vi "CANOpen_Check_Node_State.vi"(6 "Start NMT":bool, 8 "error in":errorcluster, 10 "Nodes":T2[](array[typedef]) {"NMT"."Node init static SDO state" items=["start remote node"=1, "enter pre-operational"=128]; "NMT"."Node run state" items=["start remote node"=1, "stop remote node"=2, "enter pre-operational"=128, "reset node"=129, "reset communication"=130]; "Dynamic SDOs"."Sub-Index (0)" format="%.0x"; "Dynamic SDOs"."Object Index" format="%.0x"; "Dynamic SDOs"."Block Data" format="%.0x"; "RPDOs"."PDO Channel" items=["PDO 1", "PDO 2", "PDO 3", "PDO 4"]; "RPDOs"."Parameters"."Bit Offset" max=8 step=1; "RPDOs"."Parameters"."Byte Offset" max=8 step=1; "TPDOs"."PDO Channel" items=["PDO 1", "PDO 2", "PDO 3", "PDO 4"]; "TPDOs"."Parameters"."Bit Offset" max=8 step=1; "TPDOs"."Parameters"."Byte Offset" max=8 step=1; "SDOs"."Sub-Index (0)" format="%.0x"; "SDOs"."Object Index" format="%.0x"; "SDOs"."Block Data" format="%.0x"}, 11 "interface object":refnum<k20>) -> (0 "error out":errorcluster, 2 "States":u16[](array[ring]) items=["unknown"=1, "bootup"=0, "stopped"=4, "operational"=5, "pre-operational"=127, "connection lost"=128], 3 "interface object out":refnum<k20>, 5 "Security Ref":T1)   [LabVIEW 2021, in "CANOpen Addon Engine.lvlib"]
uses:
  CANOpen Addon Engine.lvlib
  SubVIS/CANOpen_Node Message Settings.ctl
  Shared/CANOpen_PDO Settings.ctl
  Shared/CANOpen_PDO Parameter Settings.ctl
  Shared/CANOpen_PDO Data Type.ctl
  Shared/CANopen Byte Order.ctl
  Shared/CANOpen_SDO Settings.ctl
  SubVIS/CANOpen_NMT Settings.ctl
  Shared/CanOpen_NMT_Config.ctl
  Shared/CanOpen_NMT_Static detect.ctl
  CANOpen_HB_NG_EM Refs.ctl
  <vilib>/CANopenLib/CANOPEN.llb/CANopen Emergency Create.vi
  <vilib>/CANopenLib/CANOPEN.llb/CANopen SDO Create.vi
  <vilib>/CANopenLib/CANOPEN.llb/CANopen SDO Write [U16].vi
  <vilib>/CANopenLib/CANOPEN.llb/CANopen SDO Write [U8].vi
  <vilib>/CANopenLib/CANOPEN.llb/CANopen SDO Close.vi
  <vilib>/CANopenLib/CANOPEN.llb/CANopen Node Guarding Create.vi
  <vilib>/CANopenLib/CANOPEN.llb/CANopen Node Guarding State Read.vi
  <vilib>/CANopenLib/CANOPEN.llb/CANopen Heartbeat Create.vi
  <vilib>/CANopenLib/CANOPEN.llb/CANopen Heartbeat State Read.vi
  <resource>/objmgr/CANopenNodeGuard.rc
  <resource>/objmgr/CANopenHeartbeat.rc
  <resource>/objmgr/CANopenEmergency.rc
  Shared/CANOpen Addon Shared.lvlib
panel:
  out "Timestamp":timestamp
  # "LSB"
  # "MSB"
  # "LSB"
  # "MSB"
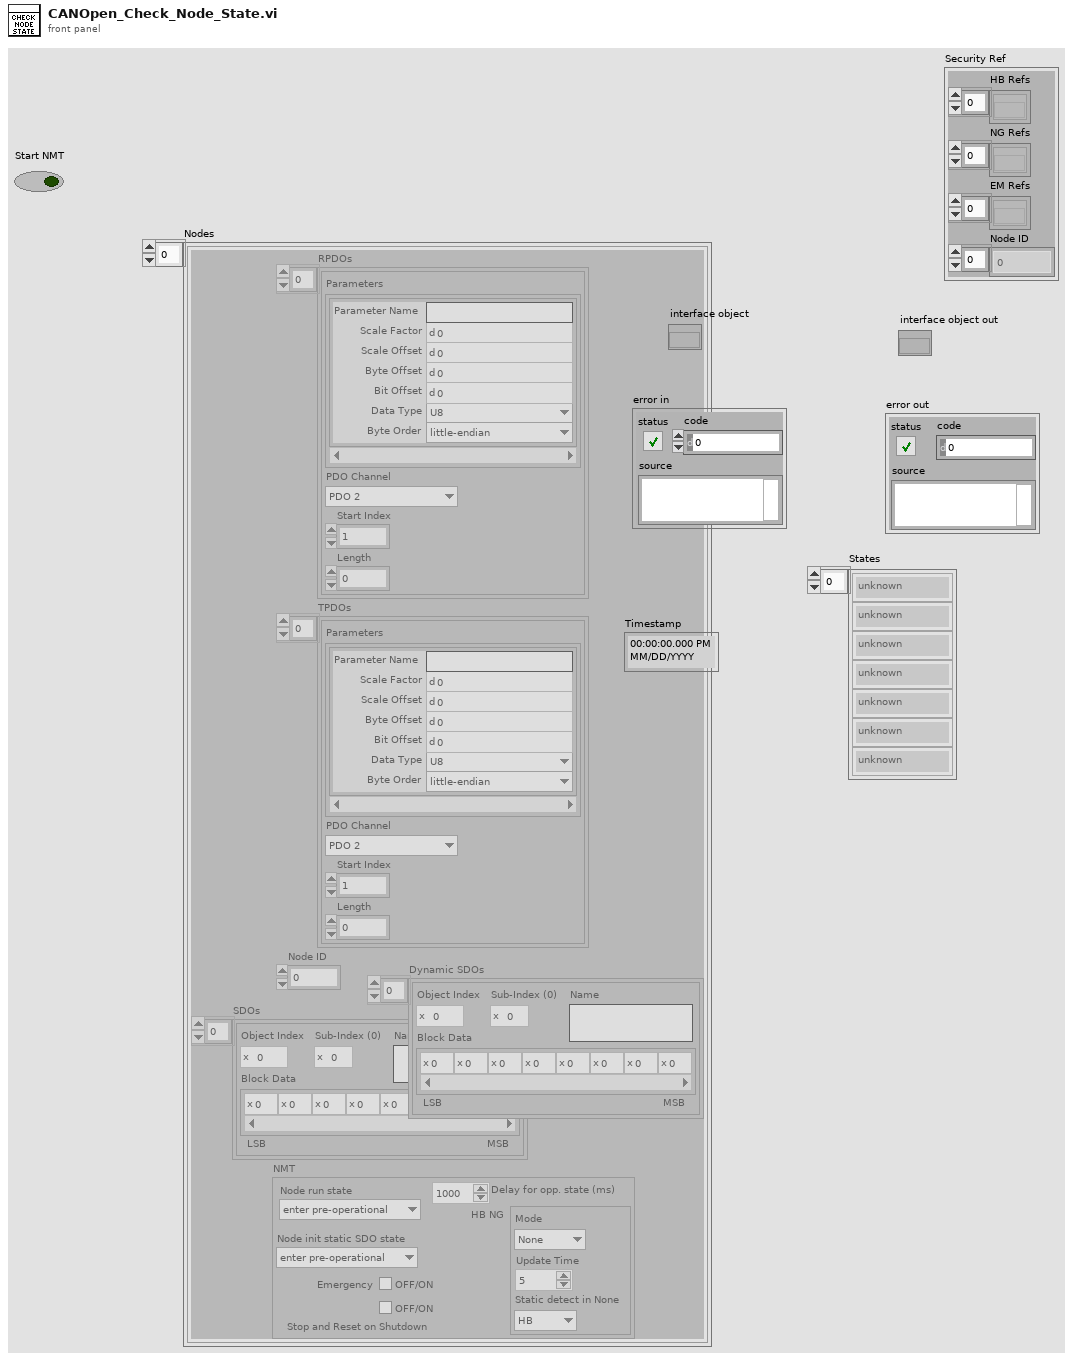
[diagram p1: front panel]
types:
  T1 = typedef "CANOpen Addon Engine.lvlib/CANOpen_HB_NG_EM Refs.ctl" = cluster{"HB Refs":refnum<k20>[], "NG Refs":refnum<k20>[], "EM Refs":refnum<k20>[], "Node ID":u8[]}
  T2 = typedef "CANOpen Addon Engine.lvlib/CANOpen_Node Message Settings.ctl" = cluster{"RPDOs":T3[], "TPDOs":T3[], "Node ID":u8, "SDOs":T7[], "Dynamic SDOs":T7[], "NMT":T8}
  T3 = typedef "CANOpen Addon Shared.lvlib/CANOpen_PDO Settings.ctl" = cluster{"Parameters":T4[], "PDO Channel":u8, "Start Index":u32, "Length":u32}
  T4 = typedef "CANOpen Addon Shared.lvlib/CANOpen_PDO Parameter Settings.ctl" = cluster{"Parameter Name":string, "Scale Factor":dbl, "Scale Offset":dbl, "Byte Offset":u8, "Bit Offset":u8, "Data Type":T5, "Byte Order":T6}
  T5 = typedef "CANOpen Addon Shared.lvlib/CANOpen_PDO Data Type.ctl" = enum16{"U8", "U16", "U32", "I8", "I16", "I32", "Single", "Double", "Boolean"}
  T6 = typedef "CANOpen Addon Shared.lvlib/CANopen Byte Order.ctl" = enum16{"big-endian network order", "little-endian"}
  T7 = typedef "CANOpen Addon Shared.lvlib/CANOpen_SDO Settings.ctl" = cluster{"Object Index":u16, "Sub-Index (0)":u8, "Block Data":u8[], "Name":string}
  T8 = typedef "CANOpen Addon Engine.lvlib/CANOpen_NMT Settings.ctl" = cluster{"Node run state":u16, "Emergency":bool, "HB NG":T9, "Delay for opp. state (ms)":dbl, "Node init static SDO state":u16, "Stop and Reset on Shutdown":bool}
  T9 = typedef "CANOpen Addon Shared.lvlib/CanOpen_NMT_Config.ctl" = cluster{"Mode":T10, "Update Time":u16, "Static detect in None":T10}
  T10 = typedef "CANOpen Addon Shared.lvlib/CanOpen_NMT_Static detect.ctl" = enum16{"None", "HB", "NG"}
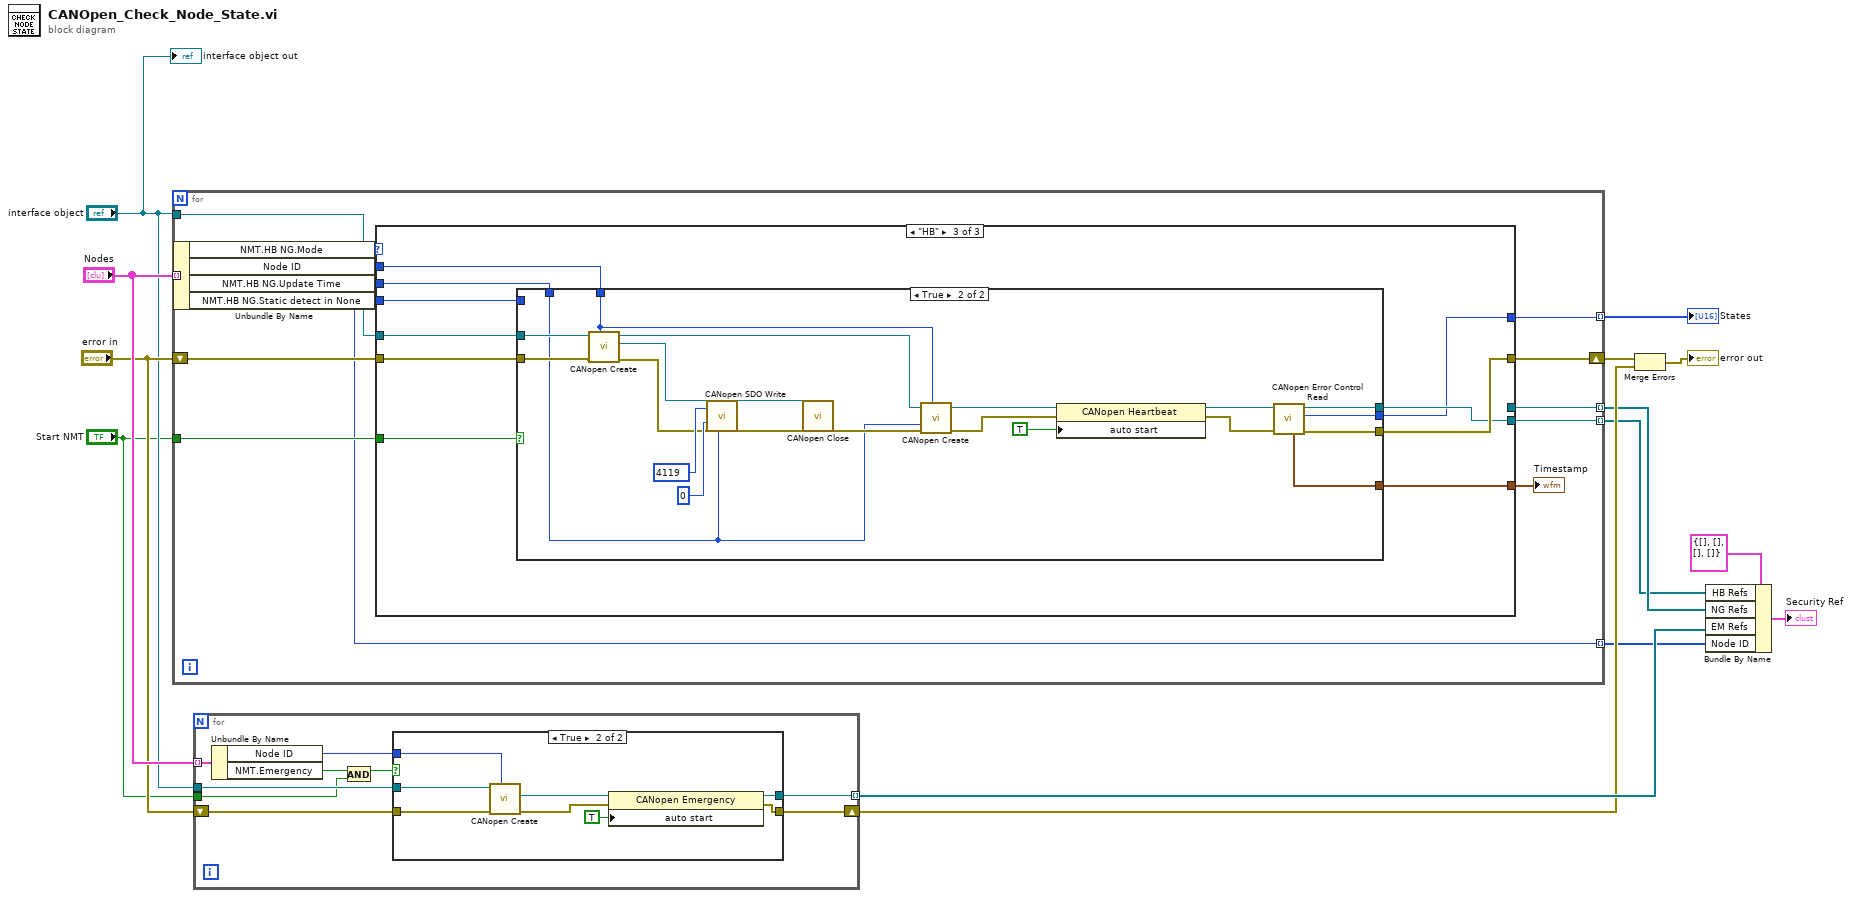
[diagram p0: block diagram]
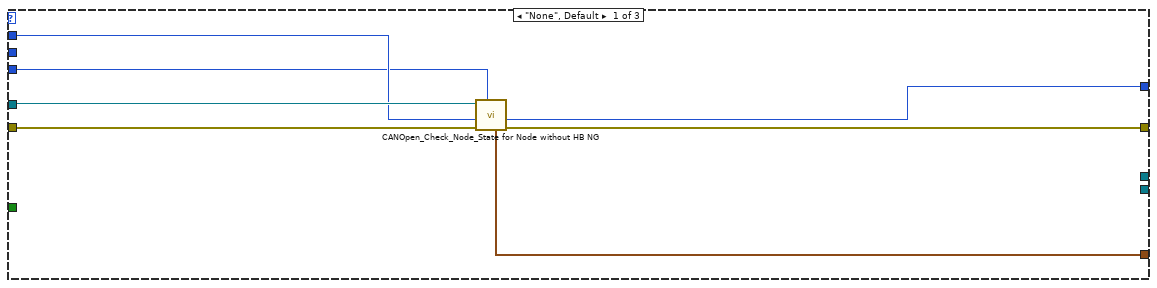
[diagram p3: hidden frame]
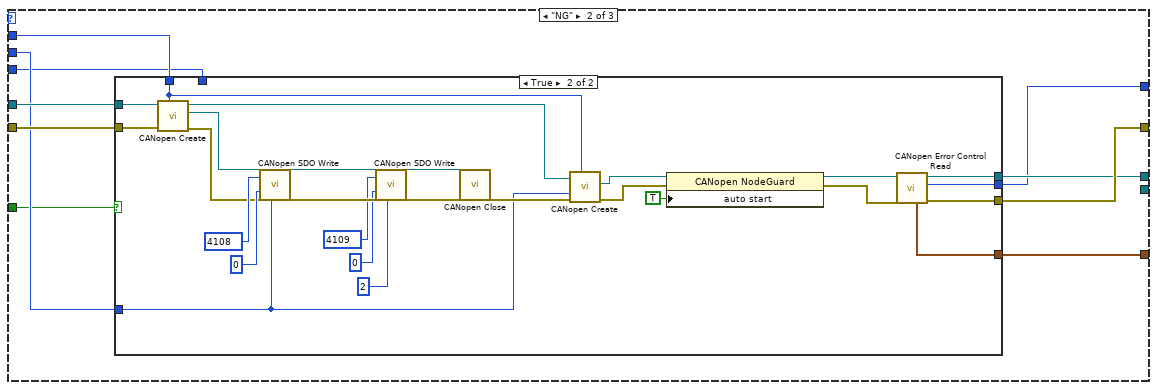
[diagram p4: hidden frame]
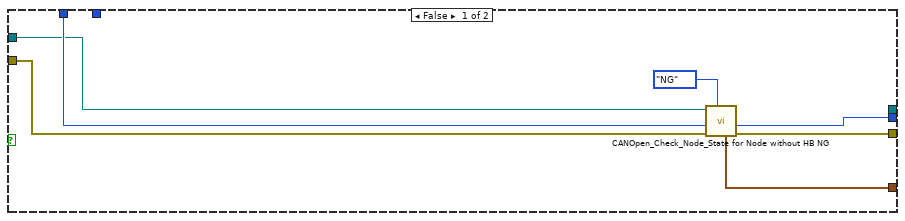
[diagram p5: hidden frame]
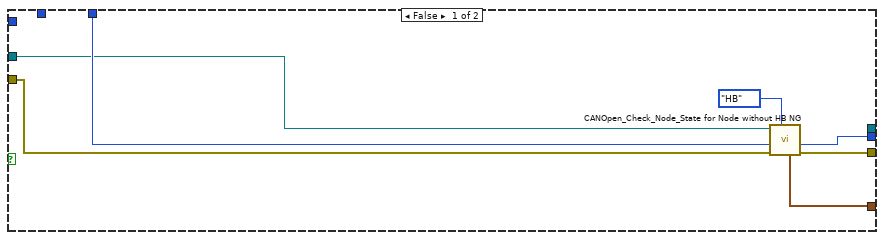
[diagram p6: hidden frame]
diagram:
  n1 = for {
    tunnel: "Nodes" -> [w27] mode=indexing
    tunnel: "interface object" -> [w26]
    shift-right: [w24] -> w14
    shift-left: "error in" -> [w19]
    tunnel: [w25] -> w13 mode=indexing
    tunnel: [w21] -> w4 mode=indexing
    tunnel: [w20] -> w3 mode=indexing
    tunnel: "Start NMT" -> [w18]
    tunnel: [w17] -> w1 mode=indexing
    n2 = Unbundle By Name(w27) -> ("NMT.HB NG.Mode"=w23:T10, "Node ID"=w17:u8, "NMT.HB NG.Update Time"=w15:u16, "NMT.HB NG.Static detect in None"=w16:T10)
    n3 = case shown="\"HB\"" w23 {
      tunnel: w19 -> [w30 w44 w87]
      tunnel: w26 -> [w34 w43 w86]
      tunnel: [w31 w37 w80] -> w25
      tunnel: [w29 w39 w82] -> w24
      tunnel: w17 -> [w33 w42 w85]
      tunnel: w15 -> [_ w41 w84]
      tunnel: [w32 w36 w79] -> w22
      tunnel: [_ w38 _] -> w21
      tunnel: [_ _ w81] -> w20
      tunnel: w18 -> [_ w40 w83]
      tunnel: w16 -> [w28 w35 w78]
      frame "None", Default {
        n4 = call "CANOpen_Check_Node_State for Node without HB NG.vi"("State detect in None"=w28, "error in"=w30, "Node ID"=w33, "interface object in"=w34) -> ("error out"=w29:errorcluster, "Last State"=w31:u16, "timestamp"=w32:timestamp)  [unwired: 4 in, 1 out]
      }
      frame "NG" {
        n5 = case shown="True" w40 {
          tunnel: w44 -> [w49 w64]
          tunnel: w43 -> [w48 w63]
          tunnel: w42 -> [w51 w62]
          tunnel: w41 -> [_ w61]
          tunnel: [_ w55] -> w38
          tunnel: [w50 w54] -> w39
          tunnel: [w47 w53] -> w37
          tunnel: [w46 w52] -> w36
          tunnel: w35 -> [_ _]
          frame False {
            n6 = call "CANOpen_Check_Node_State for Node without HB NG.vi"("State detect in None"=CanOpen_NMT_Static_detect."NG", "error in"=w49, "Node ID"=w51, "interface object in"=w48) -> ("error out"=w50:errorcluster, "Last State"=w47:u16, "timestamp"=w46:timestamp)  [unwired: 4 in, 1 out]
          }
          frame True {
            n7 = call-poly <vilib>:"CANopen Create.vi"("node-ID"=w62, "error in (no error)"=w64, "interface object in"=w63) -> ("error out"=w66:errorcluster, "SDO object out"=w65:refnum<k20>, "interface object out"=w69:refnum<k20>)  [unwired: 6 in]
            n8 = call-poly <vilib>:"CANopen SDO Write.vi"("U16 data"=w61, "error in (no error)"=w66, "object sub-index (0)"=u8 0, "object index"=u16 4108, "SDO object in"=w65) -> ("error out"=w74:errorcluster, "SDO object out"=w72:refnum<k20>)  [unwired: 4 in, 1 out]
            n9 = call-poly <vilib>:"CANopen SDO Write.vi"("U8 data"=u8 2, "error in (no error)"=w74, "object sub-index (0)"=u8 0, "object index"=u16 4109, "SDO object in"=w72) -> ("error out"=w75:errorcluster, "SDO object out"=w73:refnum<k20>)  [unwired: 4 in, 1 out]
            n10 = call-poly <vilib>:"CANopen Close.vi"("error in (no error)"=w75, "SDO object in"=w73) -> ("error out"=w76:errorcluster)  [unwired: 9 in]
            n11 = call-poly <vilib>:"CANopen Create.vi"("node-ID"=w62, "error in (no error)"=w76, "guard time [ms]"=w61, "interface object in"=w69) -> ("error out"=w60:errorcluster, "node guarding object out"=w58:refnum<k20>)  [unwired: 5 in, 1 out]
            n12 = property class="CANopen NodeGuard"(reference=w58, error in=w60, "auto start"=TRUE) -> (reference out=w57:refnum<k20>, error out=w56:errorcluster)
            n13 = call-poly <vilib>:"CANopen Error Control Read.vi"("error in (no error)"=w56, "node guarding object in"=w57) -> ("error out"=w54:errorcluster, "state"=w53:u16, "node guarding object out"=w55:refnum<k20>, "timestamp"=w52:timestamp)  [unwired: 6 in]
          }
        }
      }
      frame "HB" {
        n14 = case shown="True" w83 {
          tunnel: w87 -> [w93 w109]
          tunnel: w86 -> [w91 w108]
          tunnel: w85 -> [w92 w107]
          tunnel: w84 -> [_ w106]
          tunnel: [_ w97] -> w81
          tunnel: [w94 w98] -> w82
          tunnel: [w89 w96] -> w80
          tunnel: [w90 w95] -> w79
          tunnel: w78 -> [_ _]
          frame False {
            n15 = call "CANOpen_Check_Node_State for Node without HB NG.vi"("State detect in None"=CanOpen_NMT_Static_detect."HB", "error in"=w93, "Node ID"=w92, "interface object in"=w91) -> ("error out"=w94:errorcluster, "Last State"=w89:u16, "timestamp"=w90:timestamp)  [unwired: 4 in, 1 out]
          }
          frame True {
            n16 = call-poly <vilib>:"CANopen Create.vi"("node-ID"=w107, "error in (no error)"=w109, "interface object in"=w108) -> ("error out"=w111:errorcluster, "SDO object out"=w110:refnum<k20>, "interface object out"=w114:refnum<k20>)  [unwired: 6 in]
            n17 = call-poly <vilib>:"CANopen SDO Write.vi"("U16 data"=w106, "error in (no error)"=w111, "object sub-index (0)"=u8 0, "object index"=u16 4119, "SDO object in"=w110) -> ("error out"=w101:errorcluster, "SDO object out"=w102:refnum<k20>)  [unwired: 4 in, 1 out]
            n18 = call-poly <vilib>:"CANopen Close.vi"("error in (no error)"=w101, "SDO object in"=w102) -> ("error out"=w115:errorcluster)  [unwired: 9 in]
            n19 = call-poly <vilib>:"CANopen Create.vi"("node-ID"=w107, "error in (no error)"=w115, "consumer time [ms]"=w106, "interface object in"=w114) -> ("error out"=w104:errorcluster, "heartbeat object out"=w105:refnum<k20>)  [unwired: 5 in, 1 out]
            n20 = property class="CANopen Heartbeat"(reference=w105, error in=w104, "auto start"=TRUE) -> (reference out=w100:refnum<k20>, error out=w99:errorcluster)
            n21 = call-poly <vilib>:"CANopen Error Control Read.vi"("error in (no error)"=w99, "heartbeat object in"=w100) -> ("error out"=w98:errorcluster, "state"=w96:u16, "heartbeat object out"=w97:refnum<k20>, "timestamp"=w95:timestamp)  [unwired: 6 in]
          }
        }
      }
    }
    "Timestamp" <- w22
  }
  "States" <- w13
  n22 = for {
    tunnel: "Nodes" -> [w124] mode=indexing
    shift-right: [w119] -> w5
    shift-left: "error in" -> [w121]
    tunnel: "interface object" -> [w120]
    tunnel: [w118] -> w7 mode=indexing
    tunnel: "Start NMT" -> [w116]
    n23 = Unbundle By Name(w124) -> ("Node ID"=w122:u8, "NMT.Emergency"=w123:bool)
    n24 = And(x=w123, y=w116) -> (x .and. y?=w117:bool)
    n25 = case shown="True" w117 {
      tunnel: w122 -> [_ w133]
      tunnel: w121 -> [w125 w132]
      tunnel: w120 -> [_ w131]
      tunnel: [w125 w126] -> w119
      tunnel: [_ w129] -> w118
      frame False {
      }
      frame True {
        n26 = call-poly <vilib>:"CANopen Create.vi"("node-ID"=w133, "error in (no error)"=w132, "interface object in"=w131) -> ("error out"=w127:errorcluster, "emergency object out"=w130:refnum<k20>)  [unwired: 6 in, 1 out]
        n27 = property class="CANopen Emergency"(reference=w130, error in=w127, "auto start"=TRUE) -> (reference out=w129:refnum<k20>, error out=w126:errorcluster)
      }
    }
  }
  n28 = Merge Errors(w14, w5) -> (→"error out":errorcluster)
  n29 = Bundle By Name(cluster=T1 {"HB Refs"=[], "NG Refs"=[], "EM Refs"=[], "Node ID"=[]} ("Security Ref"), "HB Refs"=w3, "NG Refs"=w4, "EM Refs"=w7, "Node ID"=w1) -> (→"Security Ref":T1)
  "interface object out" <- "interface object"
